vi "Write.vi"(8 "error in (no error)":errorcluster, 9 "timeout_ms (-1)":i32=-1, 10 "Message":string, 11 "ConsoleWriter in":refnum<class "ConsoleWriter.lvclass">) -> (0 "error out":errorcluster, 3 "ConsoleWriter out":refnum<class "ConsoleWriter.lvclass">)   [LabVIEW 2024, in "ConsoleWriter.lvclass"]
uses:
  ConsoleWriter.lvclass
  ConsoleWriter.lvclass/ConsoleWriter.ctl
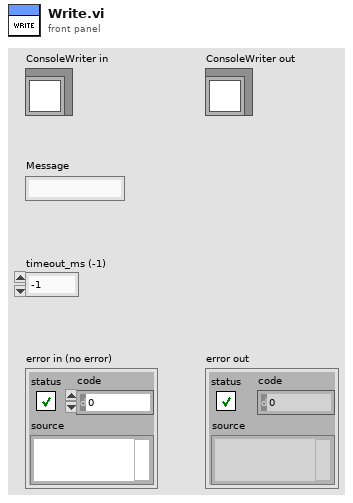
[diagram p1: front panel]
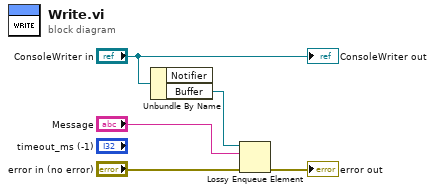
[diagram p0: block diagram]
diagram:
  n1 = Unbundle By Name("ConsoleWriter in") -> ("Buffer"=w4:refnum<queue>)  [unwired: 1 out]
  n2 = Lossy Enqueue Element(queue=w4, element="Message", error in (no error)="error in (no error)") -> (error out=→"error out":errorcluster)  [unwired: 3 out]
  "ConsoleWriter out" <- "ConsoleWriter in"
